vi "Set Default Channel Properties.vi"(7 "dt":dbl format="%#_13g", 8 "error in":errorcluster, 9 "Channel Name In":string, 10 "Group Name In":string, 11 "TDMS File In":refnum<k34>) -> (0 "error out":errorcluster, 1 "Channel Name Out":string, 2 "Group Name Out":string, 3 "TDMS File Out":refnum<k34>)   [LabVIEW 2018, in "Embedded Data Logger Engine.lvlib"]
uses:
  Embedded Data Logger Engine.lvlib
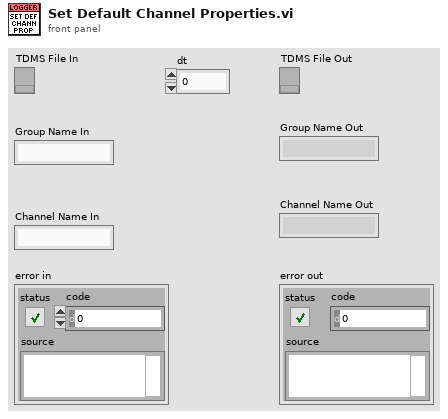
[diagram p1: front panel]
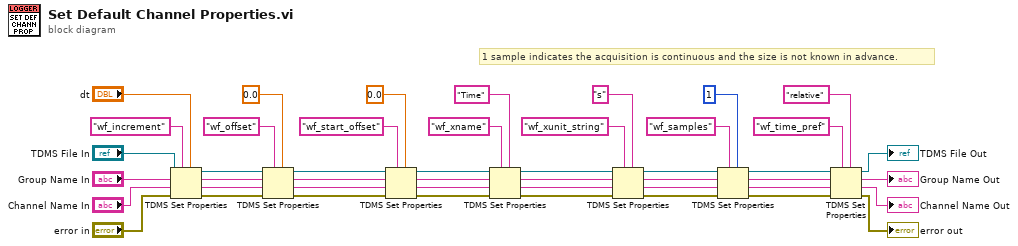
[diagram p0: block diagram]
diagram:
  # "1 sample indicates the acquisition is continuous and the size is not known in advance."
  n1 = TDMS Set Properties(5:"dt", 7:"wf_increment", 8:"error in", 9:"Channel Name In", 10:"Group Name In", 11:"TDMS File In") -> (0:w43:errorcluster, 1:w45:string, 2:w44:string, 3:w42:refnum<k34>)
  n2 = TDMS Set Properties(5:0.0 ("dt"), 7:"wf_offset", 8:w43, 9:w45, 10:w44, 11:w42) -> (0:w4:errorcluster, 1:w1:string, 2:w2:string, 3:w3:refnum<k34>)
  n3 = TDMS Set Properties(5:0.0, 7:"wf_start_offset" ("group name in (Untitled)"), 8:w4, 9:w1, 10:w2, 11:w3) -> (0:w32:errorcluster, 1:w29:string, 2:w30:string, 3:w31:refnum<k34>)
  n4 = TDMS Set Properties(5:"Time" ("group name in (Untitled)"), 7:"wf_xname" ("group name in (Untitled)"), 8:w32, 9:w29, 10:w30, 11:w31) -> (0:w25:errorcluster, 1:w21:string, 2:w22:string, 3:w26:refnum<k34>)
  n5 = TDMS Set Properties(5:"s" ("group name in (Untitled)"), 7:"wf_xunit_string" ("group name in (Untitled)"), 8:w25, 9:w21, 10:w22, 11:w26) -> (0:w19:errorcluster, 1:w13:string, 2:w14:string, 3:w20:refnum<k34>)
  n6 = TDMS Set Properties(5:1, 7:"wf_samples" ("group name in (Untitled)"), 8:w19, 9:w13, 10:w14, 11:w20) -> (0:w17:errorcluster, 1:w11:string, 2:w12:string, 3:w18:refnum<k34>)
  n7 = TDMS Set Properties(5:"relative" ("group name in (Untitled)"), 7:"wf_time_pref" ("group name in (Untitled)"), 8:w17, 9:w11, 10:w12, 11:w18) -> (0:→"error out":errorcluster, 1:→"Channel Name Out":string, 2:→"Group Name Out":string, 3:→"TDMS File Out":refnum<k34>)
